vi "Remove Subscription.vi"(8 "error in (no error)":errorcluster, 9 "Topic Filter":string, 10 "SessionMailbox":refnum<queue>, 11 "MQTT_Base in":refnum<class "MQTT_Base.lvclass">) -> (0 "error out":errorcluster, 1 "Done":bool, 3 "MQTT_Base out":refnum<class "MQTT_Base.lvclass">)   [LabVIEW 2013, in "MQTT Server.lvlib" / "MQTT_Base.lvclass"]
uses:
  MQTT_Base.lvclass
  Response -- cluster.ctl
  Control Packets/ControlPacket/ControlPacket.lvclass
  MQTT_Base.lvclass/MQTT_Base.ctl
  Server/Subscription/Subscription.lvclass/Subscription.ctl
  Server/TopicFilter/TopicFilter.lvclass/TopicFilter.ctl
  Server/Subscription/Subscription.lvclass
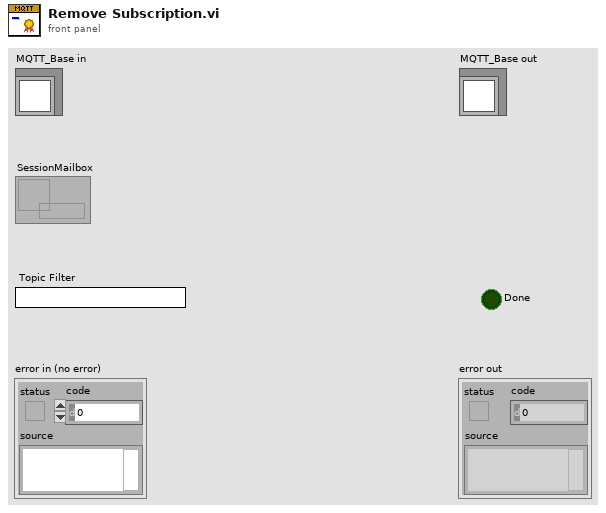
[diagram p1: front panel]
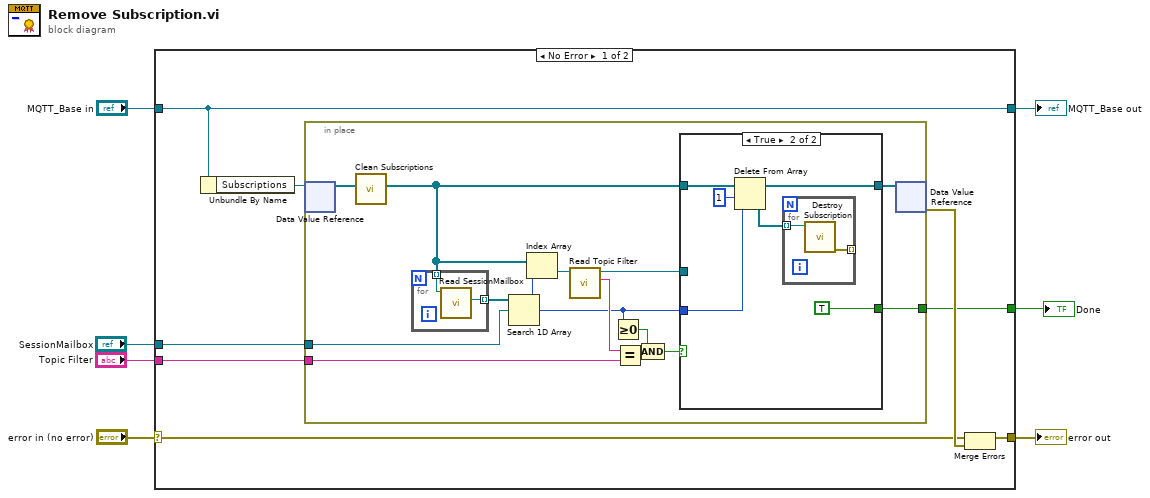
[diagram p0: block diagram]
diagram:
  n1 = case shown="No Error" "error in (no error)" {
    selector: "error in (no error)" -> [w12 w42]
    tunnel: [w11 w42] -> w6
    tunnel: [w15 w41] -> w4
    tunnel: "MQTT_Base in" -> [w15 w41]
    tunnel: "SessionMailbox" -> [w10 _]
    tunnel: [w9 _] -> w2
    tunnel: "Topic Filter" -> [w8 _]
    frame No Error {
      n2 = Unbundle By Name(w15) -> ("Subscriptions"=w14:refnum<data-value>)
      n3 = in-place {
        in-place-border: w10 -> [w28]
        in-place-border: [w20] -> w9
        in-place-border: w8 -> [w26]
        n4 = in-place-dvr #1(w14) -> (w17:refnum<class "Subscription.lvclass">[])  [unwired: 1 out]
        n5 = call "Clean Subscriptions.vi"("Subscriptions in"=w17) -> ("Subscriptions"=w16:refnum<class "Subscription.lvclass">[])  [unwired: 10 in]
        n6 = for {
          tunnel: w16 -> [w40] mode=indexing
          tunnel: [w39] -> w29 mode=indexing
          n7 = call "Read SessionMailbox.vi"("Subscription in"=w40) -> ("SessionMailbox"=w39:refnum<queue>)  [unwired: 8 in, 2 out]
        }
        n8 = Search 1D Array(1D array=w29, element=w28) -> (index of element=w21:i32)  [unwired: 1 in]
        n9 = Index Array(array=w16, index=w21) -> (element=w27:refnum<class "Subscription.lvclass">)
        n10 = call "Read Topic Filter.vi"("Subscription in"=w27) -> ("Topic Filter"=w25:string, "Subscription out"=w19:refnum<class "Subscription.lvclass">)  [unwired: 7 in, 2 out]
        n11 = Greater Or Equal To 0?(x=w21) -> (x >= 0?=w18:bool)
        n12 = Equal?(x=w25, y=w26) -> (x = y?=w24:bool)
        n13 = Compound Arithmetic op=AND(w18, w24) -> (w22:bool)
        n14 = case shown="True" w22 {
          tunnel: [w30 w34] -> w23
          tunnel: w16 -> [w30 w36]
          tunnel: w19 -> [_ _]
          tunnel: w21 -> [_ w35]
          tunnel: [_ TRUE] -> w20
          frame False {
            # "Subscription\nnot found."
          }
          frame True {
            n15 = Delete From Array(array=w36, length=1, index=w35) -> (deleted portion=w31:refnum<class "Subscription.lvclass">[], array with subset deleted=w34:refnum<class "Subscription.lvclass">[])
            n16 = for {
              tunnel: w31 -> [w38] mode=indexing
              tunnel: [w37] -> _ mode=indexing
              n17 = call "Destroy Subscription.vi"("Subscription in"=w38) -> ("error out"=w37:errorcluster)  [unwired: 9 in, 1 out]
            }
          }
        }
        n18 = in-place-dvr #1(w23) -> (w13:errorcluster)  [unwired: 1 out]
      }
      n19 = Merge Errors(w12, w13) -> (w11:errorcluster)
    }
    frame Error {
    }
  }
  "error out" <- w6
  "MQTT_Base out" <- w4
  "Done" <- w2
